vi "HasFilter.vi"(8 "error in (no error)":errorcluster, 11 "CItemMatch in":refnum<class "CItemMatch.lvclass">) -> (0 "error out":errorcluster, 1 "Has filter?":bool, 3 "CItemMatch out":refnum<class "CItemMatch.lvclass">)   [LabVIEW 2020, in "DependencyInspection.lvlib" / "CItemMatch.lvclass"]
uses:
  CItemMatch.lvclass
  TypeDefs/ComparisonType.ctl
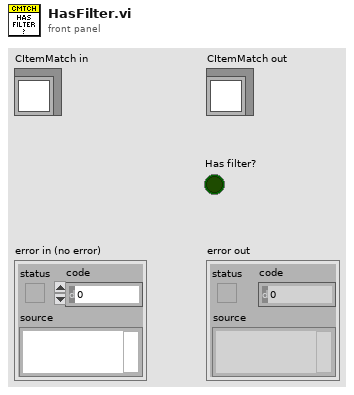
[diagram p1: front panel]
types:
  T1 = typedef "DependencyInspection.lvlib/CItemMatch.lvclass/ComparisonType.ctl" = enum16{"None", "Ends with", "Equals", "Not equal", "Starts with", "Contains", "Matches pattern"}
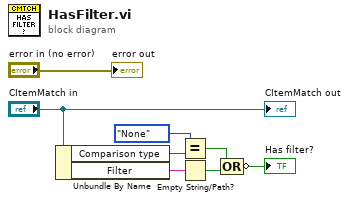
[diagram p0: block diagram]
diagram:
  n1 = Unbundle By Name("CItemMatch in") -> ("Comparison type"=w6:T1, "Filter"=w4:string)
  n2 = Equal?(x=ComparisonType."None", y=w6) -> (x = y?=w3:bool)
  n3 = Empty String/Path?(string/path=w4) -> (empty?=w2:bool)
  n4 = Compound Arithmetic op=OR(w3, w2) -> (invert →"Has filter?":bool)
  "error out" <- "error in (no error)"
  "CItemMatch out" <- "CItemMatch in"
